vi "Timer Log.vi"(10 "flag":bool, 11 "toggle":bool) -> ()   [LabVIEW 2009, in "Magnet.lvclass"]
uses:
  Magnet.lvclass
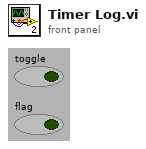
[diagram p1: front panel]
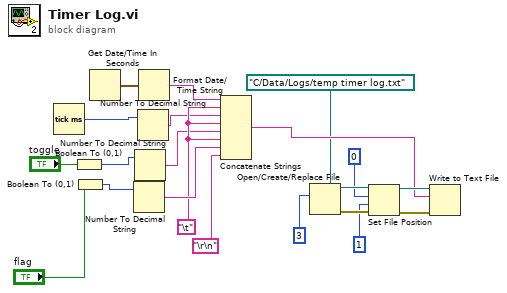
[diagram p0: block diagram]
diagram:
  w16 = "\t"
  n1 = Tick Count (ms)() -> (millisecond timer value=w20:u32)
  n2 = Boolean To (0,1)(Boolean="toggle") -> (0, 1=w12:i16)
  n3 = Boolean To (0,1)(Boolean="flag") -> (0, 1=w19:i16)
  n4 = Get Date/Time In Seconds() -> (seconds since 1Jan1904=w21:timestamp)
  n5 = Number To Decimal String(number=w19) -> (decimal integer string=w17:string)  [unwired: 1 out]
  n6 = Number To Decimal String(number=w12) -> (decimal integer string=w13:string)  [unwired: 1 out]
  n7 = Number To Decimal String(number=w20) -> (decimal integer string=w14:string)  [unwired: 1 out]
  n8 = Format Date/Time String(seconds (now)=w21) -> (date/time string=w15:string)  [unwired: 2 out]
  n9 = Concatenate Strings(w15, w16, w14, w16, w13, w16, w17, "\r\n") -> (w7:string)
  n10 = Open/Create/Replace File(file path (use dialog)=path "C:/Data/Logs/temp timer log.txt", operation (0:open)=3) -> (refnum out=w9:refnum<file>, error out=w10:errorcluster)  [unwired: 1 in, 4 out]
  n11 = Set File Position(offset (in bytes) (0)=0, refnum=w9, from (0:start)=1, error in=w10) -> (refnum out=w11:refnum<file>, error out=w8:errorcluster)
  n12 = Write to Text File(file (use dialog)=w11, text=w7, error in=w8) -> ()  [unwired: 4 out]
